vi "juke2.vi"() -> ()   [LabVIEW 2016]
doc: "This VI allows the user to select a genre of music that has preset songs that can be played for the user's pleasure. The VI will output the audio of the song as well as the waveform graph that corresponds to the audio. The user has the ability to stop a song if they please and select a new song. Also, they can change the volume of the song."
uses:
  <vilib>/sound2/lvsound2.llb/Sampling Mode.ctl
  <vilib>/sound2/lvsound2.llb/Sound File Info (path).vi
  <vilib>/sound2/lvsound2.llb/Sound File Read Open.vi
  <vilib>/sound2/lvsound2.llb/Sound File Read (DBL).vi
  <vilib>/sound2/lvsound2.llb/Sound Output Write (DBL).vi
panel:
  in  "Debug Button":bool
  in  "Initial Speed":dbl(knob)=1.0 scale=0.1..5.0 scale format="%#_2g"
  in  "Waves?":bool=TRUE
  in  "Music Location":path
  in  "Volume":dbl(knob)=1.0 scale=0.1..5.0
  in  "Cluster":T1
  in  "OK Button 2":bool
  in  "Stop":bool
  in  "stop":bool
  out "?":waveform(dbl)[](graph)
  out "String":string
  out "WARNING:":string
  out "output cluster 3":T2
  out "output cluster 2":T3
  out "output cluster":cluster{i32, i32, i32, i32, i32, i32, i32}
  # "Instructions:\nRun the program\n\nMap the Music Location to the folder that holds the files \ncontaining the music\n\nSelect a genre of music that you wish to listen to\nIf you want to select another genre, click on the genre you \nselected first. This will allow you to see a different genre. \nThen, press on the new genre you would like to listen to.\n\nSelect one of the songs. Do not select more than one song \nor an error will occur.\n\nTo play the song, press the play music button\n\nIf you wish to stop the song that is currently playing, press \nthe stop music button\n\nYou can alter the volume of the song while it is playing.\n\nYou can also alter the speed in which the song plays. However, \nyou cannot do this while the song is playing. You will have to \nstop the music from playing, alter the speed of the song, and \nthen press play music again.\n\nIf an error occurs, press the debug button to see a list of things \nthat could have potentially gone wrong.\n\nIf you do not want to see the waveform graph, press the wave\nbutton."
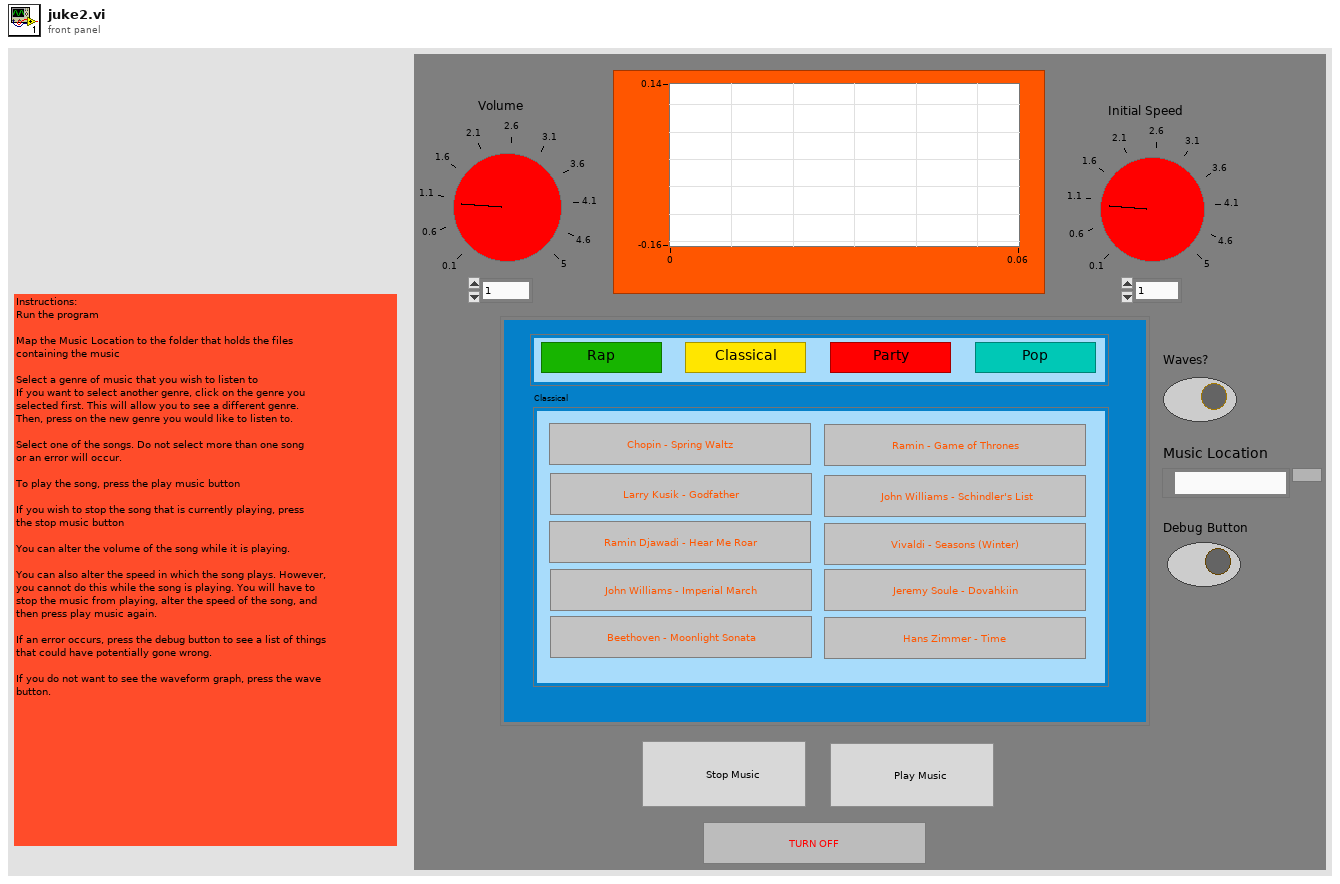
[diagram p1: front panel]
types:
  T1 = cluster{"Party":cluster{"Cazette":bool, "Steve Aoki":bool, "Imagine Dragons":bool, "Bad":bool, "boom boom pow":bool, "Make it bun dem":bool, "Cheap Thrills":bool, "She wolf":bool, "warrior":bool, "let's get it started":bool}, "Cluster 2":cluster{"OK Button":bool, "OK Button 2":bool, "OK Button 3":bool, "OK Button 4":bool}, "Rap":cluster{"Kendrick":bool, "Future":bool, "day and nite":bool, "rolex":bool, "the heart":bool, "dat new new":bool, "logic":bool, "Boujee":bool, "Bounce Back":bool, "Low Life":bool}, "Classical":cluster{"Chopin":bool, "Godfather":bool, "Hear Me Roar":bool, "Imperial March":bool, "Moonlight Sonata":bool, "game of thrones":bool, "Schindler's List":bool, "Seasons (Winter)":bool, "Skyrim":bool, "Time":bool}, "Pop":cluster{"guillotine":bool, "maybe idk":bool, "hand of god":bool, "location":bool, "bout bass":bool, "stressed out":bool, "24k":bool, "Close":bool, "Don't Let me Down":bool, "Ride":bool}}
  T2 = cluster{"appended path":path, "appended path":path, "appended path":path, "appended path":path, "appended path":path, "appended path":path, "appended path":path, "appended path":path, "appended path":path, "appended path":path, "appended path":path, "appended path":path}
  T3 = cluster{"appended path":path, "appended path":path, "appended path":path, "appended path":path, "appended path":path, "appended path":path, "appended path":path, "appended path":path, "appended path":path, "appended path":path, "appended path":path}
  T4 = cluster{"OK Button":bool, "OK Button 2":bool, "OK Button 3":bool, "OK Button 4":bool}
  T5 = cluster{"guillotine":bool, "maybe idk":bool, "hand of god":bool, "location":bool, "bout bass":bool, "stressed out":bool, "24k":bool, "Close":bool, "Don't Let me Down":bool, "Ride":bool}
  T6 = cluster{"Cazette":bool, "Steve Aoki":bool, "Imagine Dragons":bool, "Bad":bool, "boom boom pow":bool, "Make it bun dem":bool, "Cheap Thrills":bool, "She wolf":bool, "warrior":bool, "let's get it started":bool}
  T7 = cluster{"Kendrick":bool, "Future":bool, "day and nite":bool, "rolex":bool, "the heart":bool, "dat new new":bool, "logic":bool, "Boujee":bool, "Bounce Back":bool, "Low Life":bool}
  T8 = cluster{"Chopin":bool, "Godfather":bool, "Hear Me Roar":bool, "Imperial March":bool, "Moonlight Sonata":bool, "game of thrones":bool, "Schindler's List":bool, "Seasons (Winter)":bool, "Skyrim":bool, "Time":bool}
  T9 = typedef "Sampling Mode.ctl" = i32
  T10 = typedef "Sound Data Format.ctl" = cluster{"sample rate (S/s)":dbl, "number of channels":i32, "bits per sample":i32}
  T11 = typedef "Sound File Refnum.ctl" = refnum<file>
  T12 = cluster{dbl, "number of channels":i32, "bits per sample":i32}
  T13 = typedef "Sound Output Task ID.ctl" = u32
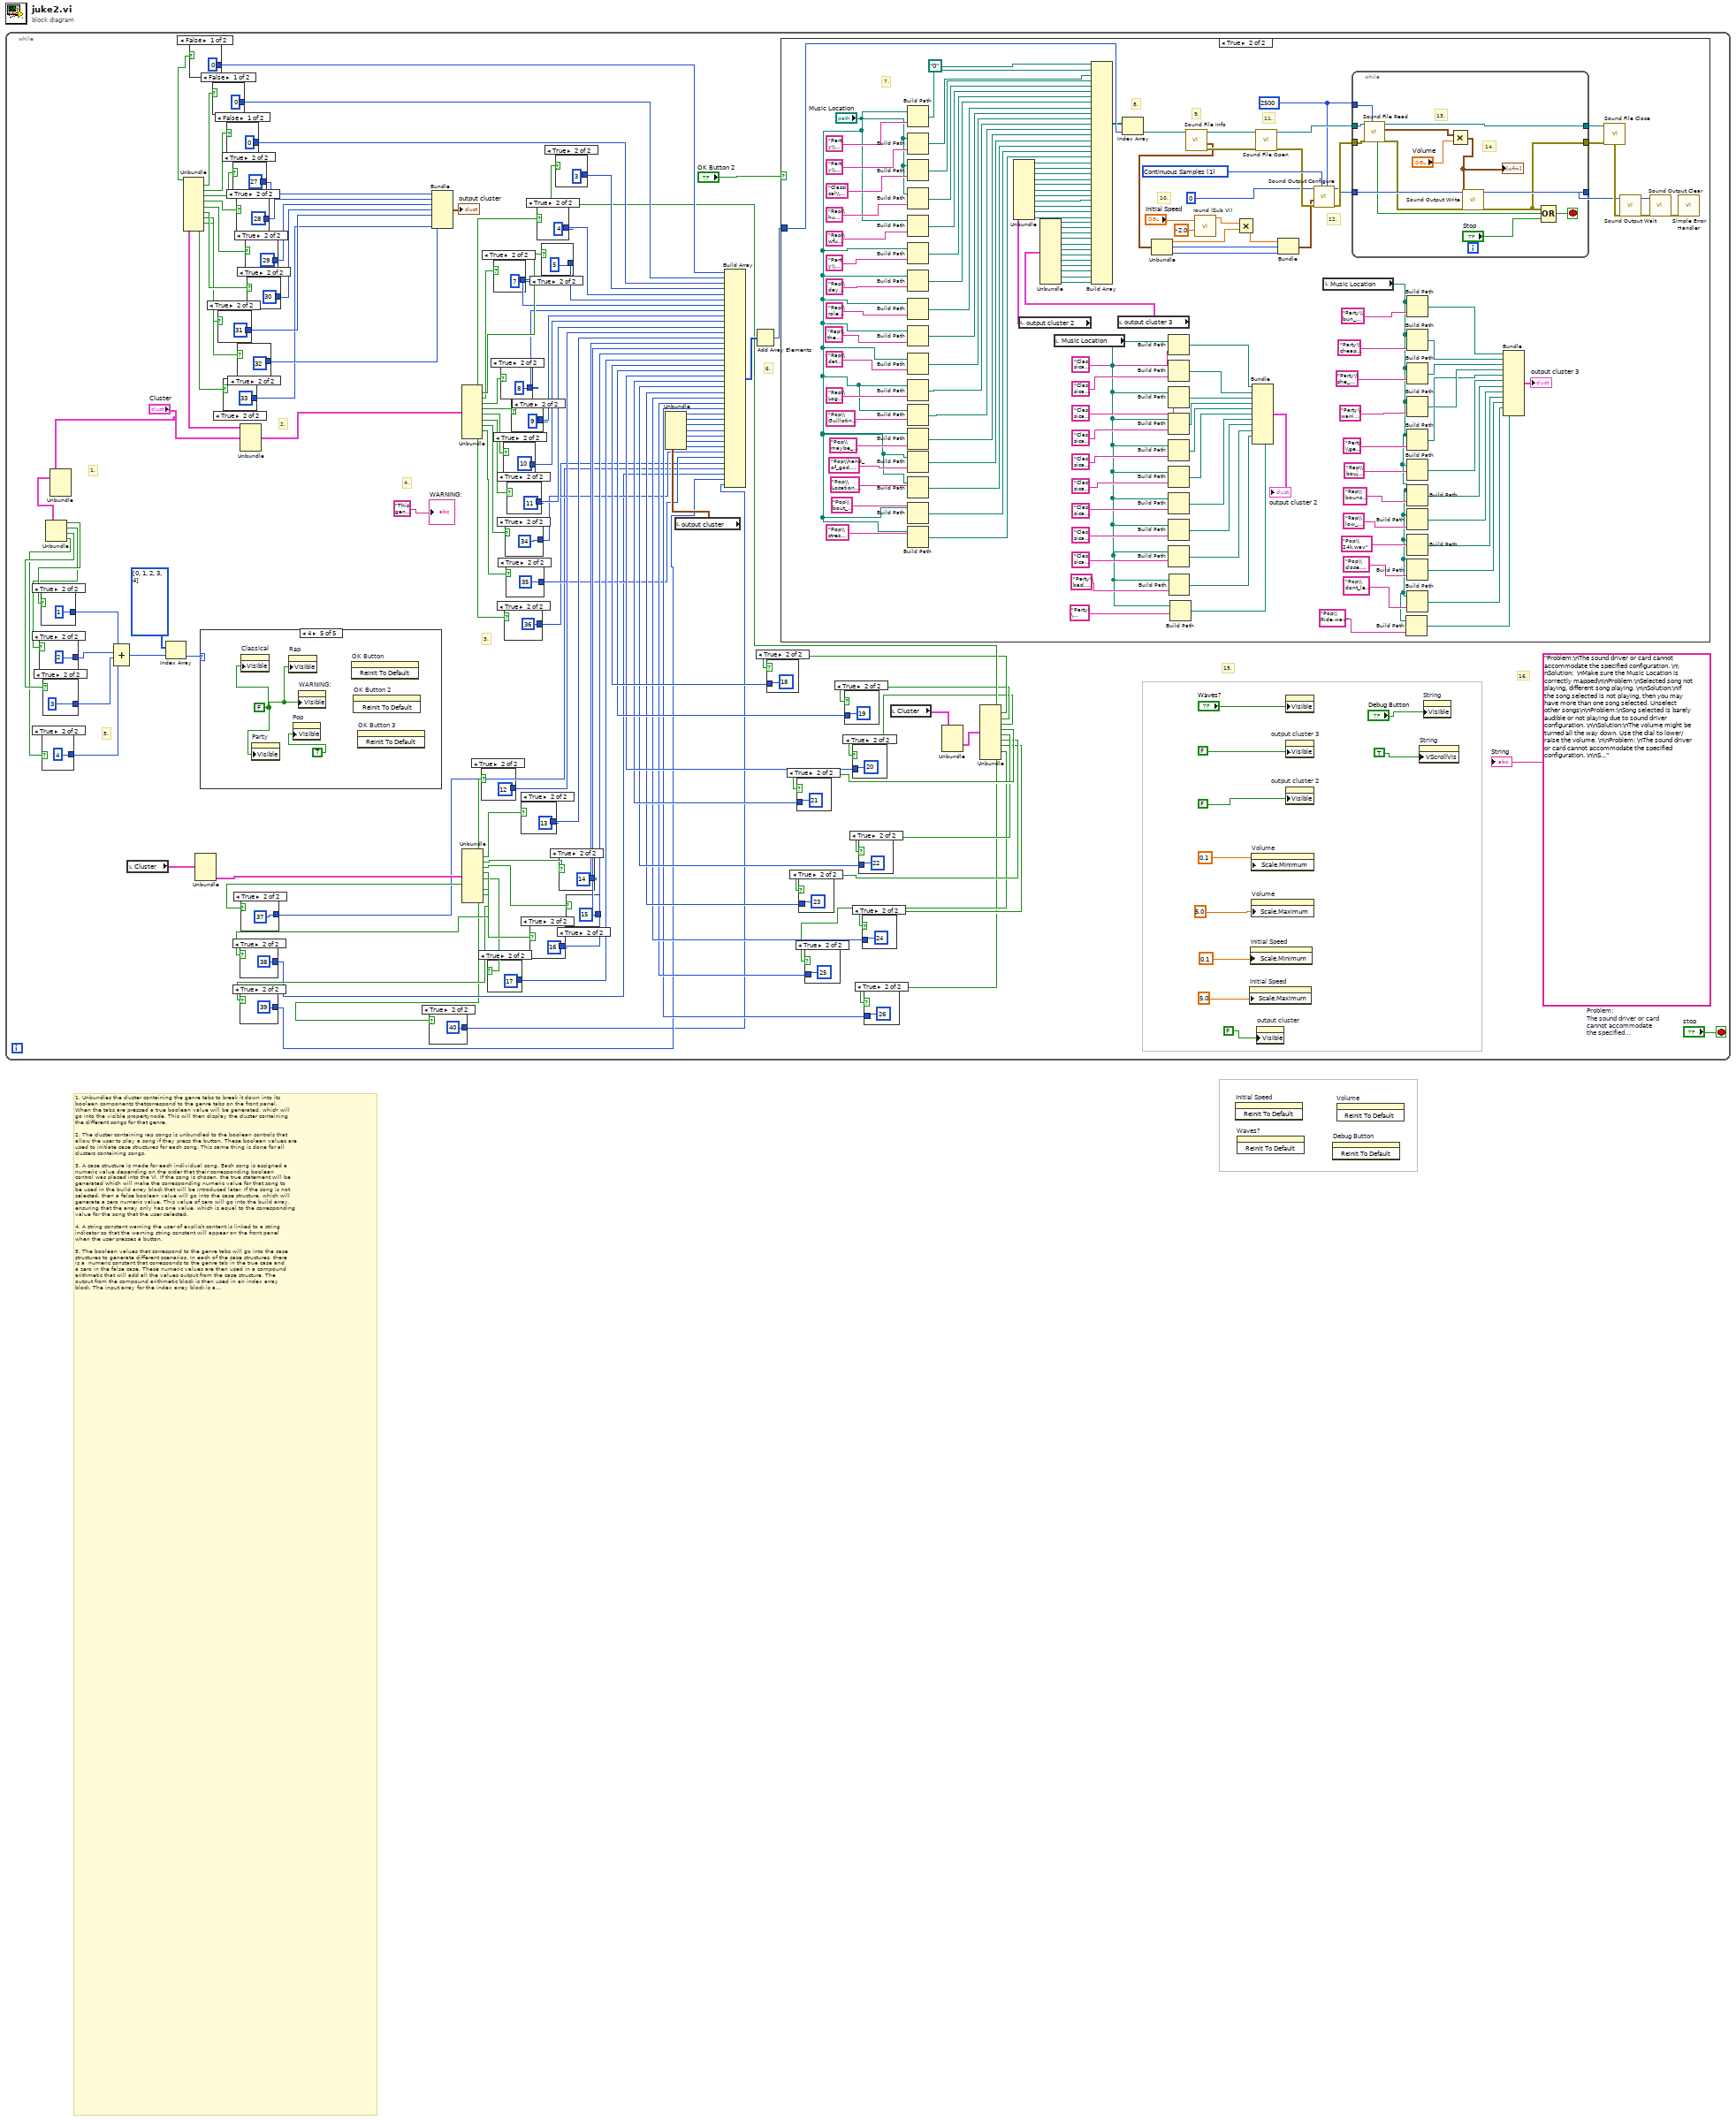
[diagram p0: block diagram]
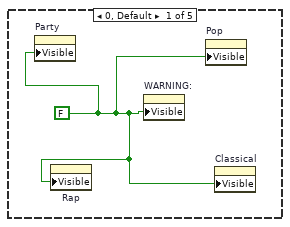
[diagram p2: hidden frame]
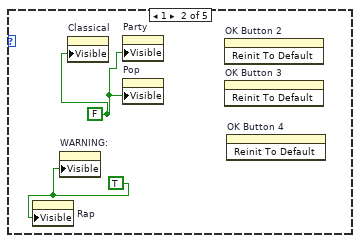
[diagram p3: hidden frame]
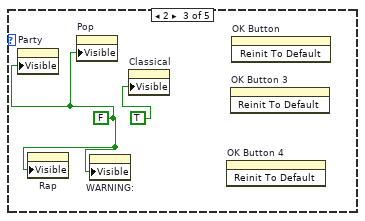
[diagram p4: hidden frame]
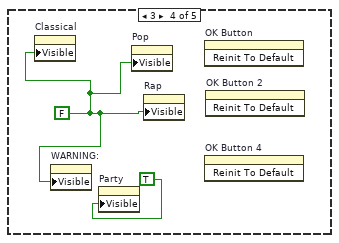
[diagram p5: hidden frame]
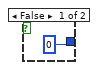
[diagram p6: hidden frame]
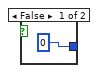
[diagram p7: hidden frame]
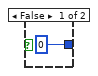
[diagram p8: hidden frame]
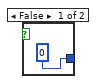
[diagram p9: hidden frame]
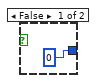
[diagram p10: hidden frame]
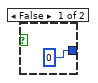
[diagram p11: hidden frame]
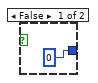
[diagram p12: hidden frame]
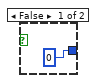
[diagram p13: hidden frame]
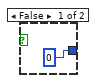
[diagram p14: hidden frame]
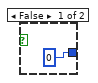
[diagram p15: hidden frame]
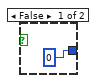
[diagram p16: hidden frame]
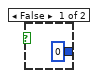
[diagram p17: hidden frame]
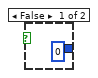
[diagram p18: hidden frame]
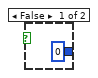
[diagram p19: hidden frame]
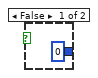
[diagram p20: hidden frame]
diagram:
  # "1. Unbundles the cluster containing the genre tabs to break it down into its \nboolean components thatcorrespond to the genre tabs on the front panel. \nWhen the tabs are pressed a true boolean value will be generated, which will \ngo into the visible propertynode. This will then display the cluster containing \nthe different songs for that genre.\n\n2. The cluster containing rap songs is unbundled to the boolean controls that\nallow the user to play a song if they press the button. These boolean values are\nused to initiate case structures for each song. This same thing is done for all\nclusters containing songs.\n\n3. A case structure is made for each individual song. Each song is assigned a \nnumeric value depending on the order that their corresponding boolean \ncontrol was placed into the VI. If the song is chosen, the true statement will be\ngenerated which will make the corresponding numeric value for that song to \nbe used in the build array block that will be introduced later. If the song is not\nselected, then a false boolean value will go into the case structure, which will \ngenerate a zero numeric value. This value of zero will go into the build array,\nensuring that the array only has one value, which is equal to the corresponding\nvalue for the song that the user selected.\n\n4. A string constant warning the user of explicit content is linked to a string \nindicator so that the warning string constant will appear on the front panel\nwhen the user presses a button.\n\n5. The boolean values that correspond to the genre tabs will go into the case \nstructures to generate different scenarios. In each of the case structures, there \nis a  numeric constant that corresponds to the genre tab in the true case and\na zero in the false case. These numeric values are then used in a compound\narithmetic that will add all the values output from the case structure. The\noutput from the compound arithmetic block is then used in an index array \nblock. The input array for the index array block is a vecotr block containing\nvalues 0-4 that correspond to the genre tab. The output from the index array\nwill go into another case structure that is defined by different numeric cases\nrather than a true and false case. In the case that a zero is input into the case,\nall of the tabs will have a false boolean value input into their Visible\nproperty node, meaning that none of the clusters showing the songs will be \ndisplayed for the user. However, depending on the case, each one will display\na different cluster that contains the songs that are under that genre.\n\n6. All  of the values that were output from the case structures are input to a \nbuild array block. Only one element in the array will contain a nonzero value. \nThis value will correspond to the song that the user selected. The array that was\nbuilt will then have all of its element values added. The output will be a single\nnumeric value that is equal to the numeric value for the song that the user \nselected.\n\n7. Each song has its own specific path that is predefined in the string constant.\nThe string constant acts as the relative path for each individual song. It is input\ninto a build path block. The base path of the songs are alsoinput into build path \nblock. This base path is defined by the user on the front panel. Each specific path \nfor each song is then input into a build array block.  Local variables are used to \norganize the block diagram. \n\n8. The array that was built in the previous step is then input into an index array\nblock. The numeric value that was outputted in step 6 that came from the \ncase structures will act as the index for the index array block. Since this numeric \nvalue corresponds to the individual song that the user selected, the value that \nwill be outut from the index array block will be the path of the song that the user\nselected.\n\n9. The specific path for the song selected goes into the Sound File Info block to\noutput the path of the song, a sound format cluster containing only numeric \nvalues, and an error out. These three outputs will be used for different things later \nin the VI.\n\n10. The sound format cluster is unbundled into three different parts. The important\npart is the sample rate because this value is multiplied by a value that will allow the\nuser to speed up or slow down the song depending on the value that they input\non the front panel.\n\n11. The path and the error out that was outputted in step 9 is then input into the \nSound File Read Open block which will open the wav file in the folder that \ncontains the song that the user selected and makes it possible for that file to be\nread.\n\n12. The Sound Output Configure block is now used to create a sound output to\ngenerate the data of the song. The inputs required for this block were constants\nand values that werw already generated. The sound format cluster that was inputted\nis the altered cluster from step 10. The sample mode was set to continuous samples\nso that the song would continue to play no matter what its duration is. The output\nfor this block is a task ID value which will be used in another block.\n\n13. The Sound File Read block is used to read the data that is inputted from the path\nthat was made to be able to read in step 11. The only things that needed to be \ninput to this block were the path of the song, the amount of samples per channel, \nand an error in value to make sure there were no errors in the VI thus far. The \nimportant outputs for this block was the data cluster, the path that at this point is\na sound file, and the error out which will be used to ensure that an error has not \noccured.\n\n14. The data cluster that is output in the previous step is multiplied by the volume \ncontrol that is on the front panel. This value is determined by the user.\n\n15.  The property nodes control the visibility of several elements. Other property \nnodes consist of setting the minimum and maximum value for the dials. The \nproperties outside the loop set the initial value for the VI when it starts. \n\n16. This is the debugging menu in which it lists out potential problems and their \nsolutions to fix the VI through small procedures,"
  n1 = while {
    stop <- "stop" stop-if-true
    w14 = "Problem:\nThe sound driver or card cannot accommodate the specified configuration. \n\nSolution:  \nMake sure the Music Location is correctly mapped\n\nProblem:\nSelected song not playing, different song playing. \n\nSolution:\nIf the song selected is not playing, then you may have more than one song selected. Unselect other songs\n\nProblem:\nSong selected is barely audible or not playing due to sound driver configuration. \n\nSolution:\nThe volume might be turned all the way down. Use the dial to lower/raise the volume. \n\nProblem: \nThe sound driver or card cannot accommodate the specified configuration. \n\nSolution: \nThe speed might be too fast or too slow for you to understand or recognize the song. Use the initial speed dial to lower/raise the speed. \n\nProblem:\nError in block diagram and function. \n\nSolution:\nRound (Sub VI) may not be in the same path as the main VI. Move main VI or other files to the same location/folder\n\nProblem: \nNo song playing in the waveform or in the VI.\n\nSolution:\nMusic Folder may not be in the same path as the main VI.  Move main VI or other files to the same location/folder. \n\nProblem:\nSelected tab not showing.\n\nSolution: \nIf one tab is not popping up, it's because another tab is open or selected.  Deselect the other tabs."  # Problem: The sound driver or card cannot accommodate the specified configuration.   Solution:   Make sure the Music Location is correctly mapped  Problem: Selected song not playing, different song playing.   Solution: If the song selected is not playing, then you may have more than one song selected. Unselect other songs  Problem: Song selected is barely audible or not playing due to sound driver configuration.   Solution: The volume might be turned all the way down. Use the dial to lower/raise the volume.   Problem:  The sound driver or card cannot accommodate the specified configuration.   Solution:  The speed might be too fast or too slow for you to understand or recognize the song. Use the initial speed dial to lower/raise the speed.   Problem: Error in block diagram and function.   Solution: Round (Sub VI) may not be in the same path as the main VI. Move main VI or other files to the same location/folder  Problem:  No song playing in the waveform or in the VI.  Solution: Music Folder may not be in the same path as the main VI.  Move main VI or other files to the same location/folder.   Problem: Selected tab not showing.  Solution:  If one tab is not popping up, it's because another tab is open or selected.  Deselect the other tabs.
    # "16."
    # "15."
    # "6."
    # "5."
    # "4."
    # "3."
    # "2."
    # "1."
    n2 = Unbundle("Cluster") -> ("Cluster 2"=w62:T4)  [unwired: 4 out]
    n3 = Unbundle(w62) -> ("OK Button"=w5:bool, "OK Button 2"=w4:bool, "OK Button 3"=w3:bool, "OK Button 4"=w2:bool)
    n4 = case shown="True" w4 {
      tunnel: [0 2] -> w11
      frame False {
      }
      frame True {
      }
    }
    n5 = case shown="True" w5 {
      tunnel: [0 1] -> w12
      frame False {
      }
      frame True {
      }
    }
    n6 = case shown="True" w2 {
      tunnel: [0 4] -> w9
      frame False {
      }
      frame True {
      }
    }
    n7 = case shown="True" w3 {
      tunnel: [0 3] -> w10
      frame False {
      }
      frame True {
      }
    }
    n8 = Compound Arithmetic op=ADD(w12, w11, w10, w9) -> (w7:i32)
    n9 = local read "Cluster"() -> (w65:T1)
    n10 = Index Array(array=i32[] [0, 1, 2, 3, 4], index=w7) -> (element=w6:i32)
    n11 = Unbundle(w65) -> ("Pop"=w64:T5)  [unwired: 4 out]
    n12 = case shown="4" w6 {
      frame 0, Default {
        w125 = FALSE
        n13 = property on="Party" class="Clust (strict)"("Visible"=w125) -> ()  [unwired: 2 in, 2 out]
        n14 = property on="Rap" class="Clust (strict)"("Visible"=w125) -> ()  [unwired: 2 in, 2 out]
        n15 = property on="WARNING:" class="Str"("Visible"=w125) -> ()  [unwired: 2 in, 2 out]
        n16 = property on="Pop" class="Clust (strict)"("Visible"=w125) -> ()  [unwired: 2 in, 2 out]
        n17 = property on="Classical" class="Clust (strict)"("Visible"=w125) -> ()  [unwired: 2 in, 2 out]
      }
      frame 1 {
        w126 = TRUE
        w127 = FALSE
        n18 = property on="Rap" class="Clust (strict)"("Visible"=w126) -> ()  [unwired: 2 in, 2 out]
        n19 = property on="WARNING:" class="Str"("Visible"=w126) -> ()  [unwired: 2 in, 2 out]
        n20 = property on="Classical" class="Clust (strict)"("Visible"=w127) -> ()  [unwired: 2 in, 2 out]
        n21 = property on="Party" class="Clust (strict)"("Visible"=w127) -> ()  [unwired: 2 in, 2 out]
        n22 = property on="Pop" class="Clust (strict)"("Visible"=w127) -> ()  [unwired: 2 in, 2 out]
        n23 = invoke on="OK Button 2" class="Bool (strict)" method="Reinit To Default"() -> ()  [unwired: 3 in, 3 out]
        n24 = invoke on="OK Button 3" class="Bool (strict)" method="Reinit To Default"() -> ()  [unwired: 3 in, 3 out]
        n25 = invoke on="OK Button 4" class="Bool (strict)" method="Reinit To Default"() -> ()  [unwired: 3 in, 3 out]
      }
      frame 2 {
        w128 = FALSE
        n26 = property on="Party" class="Clust (strict)"("Visible"=w128) -> ()  [unwired: 2 in, 2 out]
        n27 = property on="Rap" class="Clust (strict)"("Visible"=w128) -> ()  [unwired: 2 in, 2 out]
        n28 = property on="Pop" class="Clust (strict)"("Visible"=w128) -> ()  [unwired: 2 in, 2 out]
        n29 = property on="WARNING:" class="Str"("Visible"=w128) -> ()  [unwired: 2 in, 2 out]
        n30 = property on="Classical" class="Clust (strict)"("Visible"=TRUE) -> ()  [unwired: 2 in, 2 out]
        n31 = invoke on="OK Button 4" class="Bool (strict)" method="Reinit To Default"() -> ()  [unwired: 3 in, 3 out]
        n32 = invoke on="OK Button 3" class="Bool (strict)" method="Reinit To Default"() -> ()  [unwired: 3 in, 3 out]
        n33 = invoke on="OK Button" class="Bool (strict)" method="Reinit To Default"() -> ()  [unwired: 3 in, 3 out]
      }
      frame 3 {
        w130 = FALSE
        n34 = property on="Classical" class="Clust (strict)"("Visible"=w130) -> ()  [unwired: 2 in, 2 out]
        n35 = property on="WARNING:" class="Str"("Visible"=w130) -> ()  [unwired: 2 in, 2 out]
        n36 = property on="Party" class="Clust (strict)"("Visible"=TRUE) -> ()  [unwired: 2 in, 2 out]
        n37 = property on="Pop" class="Clust (strict)"("Visible"=w130) -> ()  [unwired: 2 in, 2 out]
        n38 = property on="Rap" class="Clust (strict)"("Visible"=w130) -> ()  [unwired: 2 in, 2 out]
        n39 = invoke on="OK Button" class="Bool (strict)" method="Reinit To Default"() -> ()  [unwired: 3 in, 3 out]
        n40 = invoke on="OK Button 4" class="Bool (strict)" method="Reinit To Default"() -> ()  [unwired: 3 in, 3 out]
        n41 = invoke on="OK Button 2" class="Bool (strict)" method="Reinit To Default"() -> ()  [unwired: 3 in, 3 out]
      }
      frame 4 {
        w132 = FALSE
        n42 = property on="Classical" class="Clust (strict)"("Visible"=w132) -> ()  [unwired: 2 in, 2 out]
        n43 = property on="Party" class="Clust (strict)"("Visible"=w132) -> ()  [unwired: 2 in, 2 out]
        n44 = property on="Rap" class="Clust (strict)"("Visible"=w132) -> ()  [unwired: 2 in, 2 out]
        n45 = property on="Pop" class="Clust (strict)"("Visible"=TRUE) -> ()  [unwired: 2 in, 2 out]
        n46 = property on="WARNING:" class="Str"("Visible"=w132) -> ()  [unwired: 2 in, 2 out]
        n47 = invoke on="OK Button" class="Bool (strict)" method="Reinit To Default"() -> ()  [unwired: 3 in, 3 out]
        n48 = invoke on="OK Button 2" class="Bool (strict)" method="Reinit To Default"() -> ()  [unwired: 3 in, 3 out]
        n49 = invoke on="OK Button 3" class="Bool (strict)" method="Reinit To Default"() -> ()  [unwired: 3 in, 3 out]
      }
    }
    n50 = Unbundle("Cluster") -> ("Party"=w108:T6, "Rap"=w109:T7)  [unwired: 3 out]
    n51 = Unbundle(w108) -> ("Cazette"=w110:bool, "Steve Aoki"=w114:bool, "Imagine Dragons"=w113:bool, "Bad"=w59:bool, "boom boom pow"=w58:bool, "Make it bun dem"=w53:bool, "Cheap Thrills"=w52:bool, "She wolf"=w51:bool, "warrior"=w48:bool, "let's get it started"=w36:bool)
    n52 = case shown="False" w110 {
      tunnel: [0 1] -> w122
      frame False {
      }
      frame True {
      }
    }
    n53 = case shown="False" w114 {
      tunnel: [0 2] -> w121
      frame False {
      }
      frame True {
      }
    }
    n54 = case shown="True" w51 {
      tunnel: [0 31] -> w50
      frame False {
      }
      frame True {
      }
    }
    n55 = case shown="True" w36 {
      tunnel: [0 33] -> w40
      frame False {
      }
      frame True {
      }
    }
    n56 = case shown="False" w113 {
      tunnel: [0 6] -> w120
      frame False {
      }
      frame True {
      }
    }
    n57 = case shown="True" w59 {
      tunnel: [0 27] -> w57
      frame False {
      }
      frame True {
      }
    }
    n58 = case shown="True" w58 {
      tunnel: [0 28] -> w56
      frame False {
      }
      frame True {
      }
    }
    n59 = case shown="True" w48 {
      tunnel: [0 32] -> w49
      frame False {
      }
      frame True {
      }
    }
    n60 = case shown="True" w53 {
      tunnel: [0 29] -> w55
      frame False {
      }
      frame True {
      }
    }
    n61 = case shown="True" w52 {
      tunnel: [0 30] -> w54
      frame False {
      }
      frame True {
      }
    }
    n62 = Bundle(w57, w56, w55, w54, w50, w49, w40) -> (→"output cluster":cluster{i32, i32, i32, i32, i32, i32, i32})  [unwired: 1 in]
    n63 = Unbundle(w109) -> ("Kendrick"=w111:bool, "Future"=w112:bool, "day and nite"=w106:bool, "rolex"=w104:bool, "the heart"=w103:bool, "dat new new"=w102:bool, "logic"=w101:bool, "Boujee"=w33:bool, "Bounce Back"=w34:bool, "Low Life"=w32:bool)
    n64 = Unbundle(w64) -> ("guillotine"=w94:bool, "maybe idk"=w93:bool, "hand of god"=w92:bool, "location"=w91:bool, "bout bass"=w90:bool, "stressed out"=w89:bool, "24k"=w27:bool, "Close"=w26:bool, "Don't Let me Down"=w25:bool, "Ride"=w21:bool)
    n65 = case shown="True" w26 {
      tunnel: [0 38] -> w23
      frame False {
      }
      frame True {
      }
    }
    n66 = case shown="True" w25 {
      tunnel: [0 39] -> w22
      frame False {
      }
      frame True {
      }
    }
    n67 = case shown="True" w27 {
      tunnel: [0 37] -> w24
      frame False {
      }
      frame True {
      }
    }
    n68 = case shown="True" w21 {
      tunnel: [0 40] -> w20
      frame False {
      }
      frame True {
      }
    }
    n69 = case shown="True" w94 {
      tunnel: [0 12] -> w96
      frame False {
      }
      frame True {
      }
    }
    n70 = case shown="True" w89 {
      tunnel: [0 17] -> w86
      frame False {
      }
      frame True {
      }
    }
    n71 = case shown="True" w106 {
      tunnel: [0 7] -> w105
      frame False {
      }
      frame True {
      }
    }
    n72 = case shown="True" w104 {
      tunnel: [0 8] -> w100
      frame False {
      }
      frame True {
      }
    }
    n73 = case shown="True" w102 {
      tunnel: [0 10] -> w98
      frame False {
      }
      frame True {
      }
    }
    n74 = case shown="True" w32 {
      tunnel: [0 36] -> w29
      frame False {
      }
      frame True {
      }
    }
    n75 = case shown="True" w33 {
      tunnel: [0 34] -> w31
      frame False {
      }
      frame True {
      }
    }
    n76 = case shown="True" w34 {
      tunnel: [0 35] -> w30
      frame False {
      }
      frame True {
      }
    }
    n77 = case shown="True" w101 {
      tunnel: [0 11] -> w97
      frame False {
      }
      frame True {
      }
    }
    n78 = case shown="True" w103 {
      tunnel: [0 9] -> w99
      frame False {
      }
      frame True {
      }
    }
    n79 = case shown="True" w93 {
      tunnel: [0 13] -> w81
      frame False {
      }
      frame True {
      }
    }
    n80 = case shown="True" w90 {
      tunnel: [0 16] -> w87
      frame False {
      }
      frame True {
      }
    }
    n81 = case shown="True" w111 {
      tunnel: [0 4] -> w118
      frame False {
      }
      frame True {
      }
    }
    n82 = case shown="True" w112 {
      tunnel: [0 5] -> w117
      frame False {
      }
      frame True {
      }
    }
    n83 = case shown="True" w92 {
      tunnel: [0 14] -> w95
      frame False {
      }
      frame True {
      }
    }
    n84 = case shown="True" w91 {
      tunnel: [0 15] -> w88
      frame False {
      }
      frame True {
      }
    }
    n85 = local read "output cluster"() -> (w47:cluster{i32, i32, i32, i32, i32, i32, i32})
    n86 = Unbundle(w47) -> (w46:i32, w45:i32, w44:i32, w43:i32, w42:i32, w41:i32, w35:i32)
    n87 = local read "Cluster"() -> (w61:T1)
    n88 = Unbundle(w61) -> ("Classical"=w60:T8)  [unwired: 4 out]
    n89 = Unbundle(w60) -> ("Chopin"=w107:bool, "Godfather"=w85:bool, "Hear Me Roar"=w80:bool, "Imperial March"=w79:bool, "Moonlight Sonata"=w78:bool, "game of thrones"=w76:bool, "Schindler's List"=w74:bool, "Seasons (Winter)"=w71:bool, "Skyrim"=w70:bool, "Time"=w68:bool)
    n90 = case shown="True" w107 {
      tunnel: [0 3] -> w119
      frame False {
      }
      frame True {
      }
    }
    n91 = case shown="True" w85 {
      tunnel: [0 18] -> w84
      frame False {
      }
      frame True {
      }
    }
    n92 = case shown="True" w78 {
      tunnel: [0 21] -> w77
      frame False {
      }
      frame True {
      }
    }
    n93 = case shown="True" w74 {
      tunnel: [0 23] -> w73
      frame False {
      }
      frame True {
      }
    }
    n94 = case shown="True" w70 {
      tunnel: [0 25] -> w69
      frame False {
      }
      frame True {
      }
    }
    n95 = case shown="True" w80 {
      tunnel: [0 19] -> w83
      frame False {
      }
      frame True {
      }
    }
    n96 = case shown="True" w79 {
      tunnel: [0 20] -> w82
      frame False {
      }
      frame True {
      }
    }
    n97 = case shown="True" w76 {
      tunnel: [0 22] -> w75
      frame False {
      }
      frame True {
      }
    }
    n98 = case shown="True" w71 {
      tunnel: [0 24] -> w72
      frame False {
      }
      frame True {
      }
    }
    n99 = case shown="True" w68 {
      tunnel: [0 26] -> w67
      frame False {
      }
      frame True {
      }
    }
    n100 = Build Array(w122, w121, w120, w119, w118, w117, w105, w100, w99, w98, w97, w96, w81, w95, w88, w87, w86, w84, w83, w82, w77, w75, w73, w72, w69, w67, w46, w45, w44, w43, w42, w41, w35, w31, w30, w29, w24, w23, w22, w20) -> (w116:i32[])
    n101 = Add Array Elements(numeric array=w116) -> (sum=w115:i32)
    n102 = case shown="True" "OK Button 2" {
      tunnel: w115 -> [_ w343]
      frame False {
      }
      frame True {
        w346 = 2500
        w359 = T9 1 items=["Finite Samples", "Continuous Samples"] ("sample mode")
        # "12."
        # "11."
        # "10."
        # "9."
        # "8."
        # "7."
        n103 = Build Path(base path="Music Location", name or relative path="Party\\cazette.wav") -> (appended path=w341:path)
        n104 = Build Path(base path="Music Location", name or relative path="Party\\steve_aoki.wav") -> (appended path=w340:path)
        n105 = Build Path(base path="Music Location", name or relative path="Classical\\spring_waltz.wav") -> (appended path=w339:path)
        n106 = Build Path(base path="Music Location", name or relative path="Rap\\humble.wav") -> (appended path=w338:path)
        n107 = Build Path(base path="Music Location", name or relative path="Rap\\wfuture.wav") -> (appended path=w337:path)
        n108 = Build Path(base path="Music Location", name or relative path="Party\\believer.wav") -> (appended path=w336:path)
        n109 = Build Path(base path="Music Location", name or relative path="Rap\\day_nite.wav") -> (appended path=w335:path)
        n110 = Build Path(base path="Music Location", name or relative path="Rap\\rolex.wav") -> (appended path=w334:path)
        n111 = Build Path(base path="Music Location", name or relative path="Rap\\the_heart.wav") -> (appended path=w333:path)
        n112 = Build Path(base path="Music Location", name or relative path="Rap\\dat_new_new.wav") -> (appended path=w332:path)
        n113 = Build Path(base path="Music Location", name or relative path="Rap\\Logic.wav") -> (appended path=w320:path)
        n114 = Build Path(base path="Music Location", name or relative path="Pop\\Guillotine.wav") -> (appended path=w319:path)
        n115 = Build Path(base path="Music Location", name or relative path="Pop\\maybe_idk.wav") -> (appended path=w318:path)
        n116 = Build Path(base path="Music Location", name or relative path="Pop\\hand_of_god.wav") -> (appended path=w317:path)
        n117 = Build Path(base path="Music Location", name or relative path="Pop\\Location.wav") -> (appended path=w316:path)
        n118 = Build Path(base path="Music Location", name or relative path="Pop\\bout_bass.wav") -> (appended path=w315:path)
        n119 = Build Path(base path="Music Location", name or relative path="Pop\\stressed_out.wav") -> (appended path=w308:path)
        n120 = local read "output cluster 2"() -> (w276:T3)
        n121 = Unbundle(w276) -> ("appended path"=w275:path, "appended path"=w274:path, "appended path"=w273:path, "appended path"=w272:path, "appended path"=w271:path, "appended path"=w270:path, "appended path"=w269:path, "appended path"=w268:path, "appended path"=w267:path, "appended path"=w266:path, "appended path"=w265:path)
        n122 = local read "Music Location"() -> (w295:path)
        n123 = local read "output cluster 3"() -> (w243:T2)
        n124 = Unbundle(w243) -> ("appended path"=w242:path, "appended path"=w241:path, "appended path"=w240:path, "appended path"=w239:path, "appended path"=w238:path, "appended path"=w237:path, "appended path"=w236:path, "appended path"=w235:path, "appended path"=w234:path, "appended path"=w233:path, "appended path"=w232:path, "appended path"=w231:path)
        n125 = Build Array(path "0", w341, w340, w339, w338, w337, w336, w335, w334, w333, w332, w320, w319, w318, w317, w316, w315, w308, w275, w274, w273, w272, w271, w270, w269, w268, w267, w266, w265, w242, w241, w240, w239, w238, w237, w236, w235, w234, w233, w232, w231) -> (w342:path[])
        n126 = Index Array(array=w342, index=w343) -> (element=w344:path)
        n127 = Build Path(base path=w295, name or relative path="Classical\\godfather.wav") -> (appended path=w288:path)
        n128 = Build Path(base path=w295, name or relative path="Classical\\hear_me_roar.wav") -> (appended path=w287:path)
        n129 = Build Path(base path=w295, name or relative path="Classical\\imperial_march.wav") -> (appended path=w286:path)
        n130 = Build Path(base path=w295, name or relative path="Classical\\moonlight_sonata.wav") -> (appended path=w285:path)
        n131 = Build Path(base path=w295, name or relative path="Classical\\GoT.wav") -> (appended path=w284:path)
        n132 = Build Path(base path=w295, name or relative path="Classical\\schindler.wav") -> (appended path=w283:path)
        n133 = Build Path(base path=w295, name or relative path="Classical\\seasons_winter.wav") -> (appended path=w282:path)
        n134 = Build Path(base path=w295, name or relative path="Classical\\Skyrim.wav") -> (appended path=w281:path)
        n135 = Build Path(base path=w295, name or relative path="Classical\\Time.wav") -> (appended path=w280:path)
        n136 = Build Path(base path=w295, name or relative path="Party\\bad.wav") -> (appended path=w279:path)
        n137 = Build Path(base path=w295, name or relative path="Party\\boom_boom_pow.wav") -> (appended path=w278:path)
        n138 = call-poly <vilib>:"Sound File Info.vi"("path"=w344) -> ("error out"=w351:errorcluster, "sound format"=w230:T10, "path out"=w358:path)  [unwired: 7 in, 1 out]
        n139 = Unbundle(w230) -> ("sample rate (S/s)"=w226:dbl, "number of channels"=w229:i32, "bits per sample"=w227:i32)
        n140 = call "round (Sub VI).vi"("Numeric"=-2.0, "Number to round"="Initial Speed") -> ("Rounded number"=w222:dbl)  [unwired: 9 in]
        n141 = Multiply(x=w222, y=w226) -> (x*y=w225:dbl)
        n142 = Bundle("appended path"=w288, "appended path"=w287, "appended path"=w286, "appended path"=w285, "appended path"=w284, "appended path"=w283, "appended path"=w282, "appended path"=w281, "appended path"=w280, "appended path"=w279, "appended path"=w278) -> (→"output cluster 2":T3)  [unwired: 1 in]
        n143 = call-poly <vilib>:"Sound File Open.vi"("error in (no error)"=w351, "path"=w358) -> ("error out"=w352:errorcluster, "sound file refnum"=w350:T11)  [unwired: 8 in]
        n144 = Bundle(w225, "number of channels"=w229, "bits per sample"=w227) -> (w228:T12)  [unwired: 1 in]
        n145 = call <vilib>:"Sound Output Configure.vi"("number of samples/ch"=w346, "sample mode"=w359, "error in (no error)"=w352, "sound format"=w228, "device ID"=0) -> ("error out"=w353:errorcluster, "task ID"=w347:T13)  [unwired: 5 in]
        n146 = local read "Music Location"() -> (w246:path)
        n147 = while {
          tunnel: w350 -> [w372]
          tunnel: [w371] -> w348
          tunnel: w353 -> [w373]
          tunnel: [w366] -> w349
          tunnel: w347 -> [w370]
          tunnel: [w374] -> w355
          tunnel: w346 -> [w365]
          stop <- w364 stop-if-true
          # "14."
          # "13."
          n148 = call-poly <vilib>:"Sound File Read.vi"("number of samples/ch (-1: all)"=w365, "error in (no error)"=w373, "sound file refnum"=w372) -> ("error out"=w369:errorcluster, "data"=w363:waveform(dbl)[], "sound file refnum out"=w371:T11, "end of file?"=w367:bool)  [unwired: 4 in, 1 out]
          n149 = Multiply(x=w363, y="Volume") -> (x*y=w362:waveform(dbl)[])
          "?" <- w362
          n150 = call-poly <vilib>:"Sound Output Write.vi"("error in (no error)"=w369, "data"=w362, "task ID"=w370) -> ("error out"=w366:errorcluster, "task ID out"=w374:T13)  [unwired: 7 in]
          n151 = Compound Arithmetic op=OR(w366, w367, "Stop") -> (w364:bool)
        }
        n152 = Build Path(base path=w246, name or relative path="Pop\\Ride.wav") -> (appended path=w245:path)
        n153 = Build Path(base path=w246, name or relative path="Party\\bun_dem.wav") -> (appended path=w264:path)
        n154 = Build Path(base path=w246, name or relative path="Party\\cheap_thrills.wav") -> (appended path=w263:path)
        n155 = Build Path(base path=w246, name or relative path="Party\\she_wolf.wav") -> (appended path=w262:path)
        n156 = Build Path(base path=w246, name or relative path="Party\\warrior.wav") -> (appended path=w261:path)
        n157 = Build Path(base path=w246, name or relative path="Party\\get_it_started.wav") -> (appended path=w260:path)
        n158 = Build Path(base path=w246, name or relative path="Rap\\boujee.wav") -> (appended path=w253:path)
        n159 = Build Path(base path=w246, name or relative path="Rap\\bounce_back.wav") -> (appended path=w252:path)
        n160 = Build Path(base path=w246, name or relative path="Rap\\low_life.wav") -> (appended path=w251:path)
        n161 = Build Path(base path=w246, name or relative path="Pop\\24k.wav") -> (appended path=w250:path)
        n162 = Build Path(base path=w246, name or relative path="Pop\\close.wav") -> (appended path=w249:path)
        n163 = Build Path(base path=w246, name or relative path="Pop\\dont_let_me_down.wav") -> (appended path=w248:path)
        n164 = Bundle("appended path"=w264, "appended path"=w263, "appended path"=w262, "appended path"=w261, "appended path"=w260, "appended path"=w253, "appended path"=w252, "appended path"=w251, "appended path"=w250, "appended path"=w249, "appended path"=w248, "appended path"=w245) -> (→"output cluster 3":T2)  [unwired: 1 in]
        n165 = call <vilib>:"Sound File Close.vi"("error in (no error)"=w349, "sound file refnum"=w348) -> ("error out"=w356:errorcluster)  [unwired: 9 in]
        n166 = call <vilib>:"Sound Output Wait.vi"("error in (no error)"=w356, "task ID"=w355) -> ("error out"=w357:errorcluster, "task ID out"=w354:T13)  [unwired: 8 in]
        n167 = call <vilib>:"Sound Output Clear.vi"("error in (no error)"=w357, "task ID"=w354) -> ("error out"=w360:errorcluster)  [unwired: 9 in]
        n168 = call <vilib>:"Simple Error Handler.vi"("error in (no error)"=w360) -> ()  [unwired: 4 in, 5 out]
      }
    }
    n169 = property on="Initial Speed" class="Knob (strict)"("Scale.Maximum"=5.0) -> ()  [unwired: 2 in, 2 out]
    n170 = property on="Initial Speed" class="Knob (strict)"("Scale.Minimum"=0.1) -> ()  [unwired: 2 in, 2 out]
    n171 = property on="Volume" class="Knob (strict)"("Scale.Minimum"=0.1) -> ()  [unwired: 2 in, 2 out]
    n172 = property on="Volume" class="Knob (strict)"("Scale.Maximum"=5.0) -> ()  [unwired: 2 in, 2 out]
    n173 = property on="output cluster" class="Clust (strict)"("Visible"=FALSE) -> ()  [unwired: 2 in, 2 out]
    n174 = property class="WFGraph (strict)"("Visible"="Waves?") -> ()  [unwired: 2 in, 2 out]
    n175 = property on="output cluster 3" class="Clust (strict)"("Visible"=FALSE) -> ()  [unwired: 2 in, 2 out]
    n176 = property on="output cluster 2" class="Clust (strict)"("Visible"=FALSE) -> ()  [unwired: 2 in, 2 out]
    n177 = property on="String" class="Str"("VScrollVis"=TRUE) -> ()  [unwired: 2 in, 2 out]
    n178 = property on="String" class="Str"("Visible"="Debug Button") -> ()  [unwired: 2 in, 2 out]
    "WARNING:" <- "This genre contains explicit content"
    "String" <- w14
  }
  n179 = invoke on="Initial Speed" class="Knob (strict)" method="Reinit To Default"() -> ()  [unwired: 3 in, 3 out]
  n180 = invoke on="Waves?" class="Bool (strict)" method="Reinit To Default"() -> ()  [unwired: 3 in, 3 out]
  n181 = invoke on="Debug Button" class="Bool (strict)" method="Reinit To Default"() -> ()  [unwired: 3 in, 3 out]
  n182 = invoke on="Volume" class="Knob (strict)" method="Reinit To Default"() -> ()  [unwired: 3 in, 3 out]
